vi "AerotechStateTransition.vi"(0 "error in (no error)":errorcluster, 5 "Command":T2, 7 "State In":T1) -> (3 "error out":errorcluster, 6 "Transition?":bool, 10 "State Out":T1)   [LabVIEW 2009]
uses:
  Controls/AerotechState.ctl
  Controls/AerotechCommand.ctl
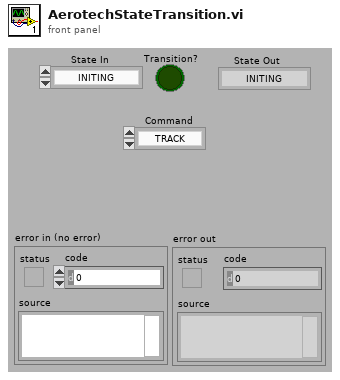
[diagram p1: front panel]
types:
  T1 = typedef "AerotechState.ctl" = enum16{"INITING", "IDLING", "SLEWING", "TRACKING", "MOVING", "HOMING", "STOPPING", "RECORDING"}
  T2 = typedef "AerotechCommand.ctl" = enum16{"TRACK", "POSITION", "STOP", "HOME", "QUIT", "RECORD"}
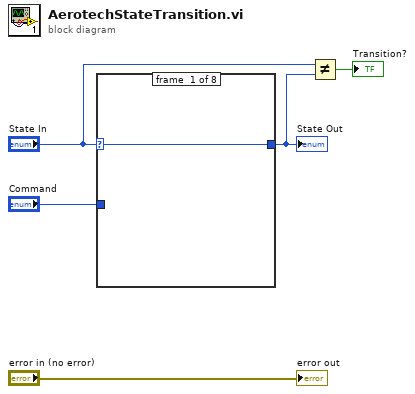
[diagram p0: block diagram]
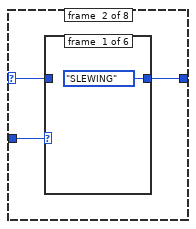
[diagram p2: hidden frame]
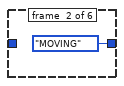
[diagram p3: hidden frame]
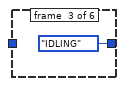
[diagram p4: hidden frame]
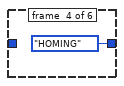
[diagram p5: hidden frame]
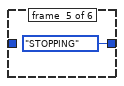
[diagram p6: hidden frame]
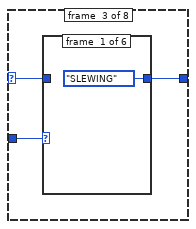
[diagram p8: hidden frame]
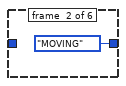
[diagram p9: hidden frame]
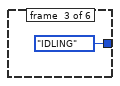
[diagram p10: hidden frame]
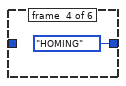
[diagram p11: hidden frame]
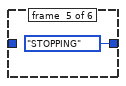
[diagram p12: hidden frame]
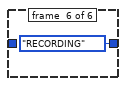
[diagram p13: hidden frame]
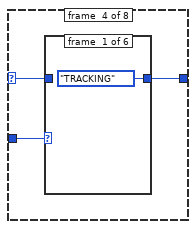
[diagram p14: hidden frame]
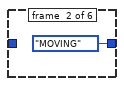
[diagram p15: hidden frame]
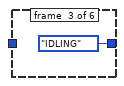
[diagram p16: hidden frame]
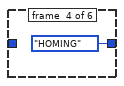
[diagram p17: hidden frame]
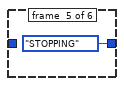
[diagram p18: hidden frame]
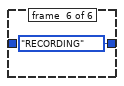
[diagram p19: hidden frame]
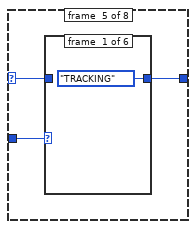
[diagram p20: hidden frame]
diagram:
  n1 = case shown="\"SLEWING\"" "State In" {
    selector: "State In" -> [w6 w7 w17 w26 w35 w44 w52 w53]
    tunnel: "Command" -> [_ w9 w18 w27 w36 w45 _ _]
    tunnel: [w6 w8 w16 w25 w34 w43 w52 w53] -> w3
    frame #0 {
    }
    frame #1 {
      n2 = case shown="\"TRACK\", Default" w9 {
        tunnel: [AerotechState."SLEWING" ("State In") AerotechState."MOVING" ("State In") AerotechState."IDLING" ("State In") AerotechState."HOMING" ("State In") AerotechState."STOPPING" ("State In") w15] -> w8
        tunnel: w7 -> [_ _ _ _ _ w15]
        frame #0 {
        }
        frame #1 {
        }
        frame #2 {
        }
        frame #3 {
        }
        frame #4 {
        }
        frame #5 {
        }
      }
    }
    frame #2 {
      n3 = case shown="\"RECORD\"" w18 {
        tunnel: w17 -> [_ _ _ _ _ _]
        tunnel: [AerotechState."SLEWING" ("State In") AerotechState."MOVING" ("State In") AerotechState."IDLING" ("State In") AerotechState."HOMING" ("State In") AerotechState."STOPPING" ("State In") AerotechState."RECORDING" ("State In")] -> w16
        frame #0 {
        }
        frame #1 {
        }
        frame #2 {
        }
        frame #3 {
        }
        frame #4 {
        }
        frame #5 {
        }
      }
    }
    frame #3 {
      n4 = case shown="\"RECORD\"" w27 {
        tunnel: w26 -> [_ _ _ _ _ _]
        tunnel: [AerotechState."TRACKING" ("State In") AerotechState."MOVING" ("State In") AerotechState."IDLING" ("State In") AerotechState."HOMING" ("State In") AerotechState."STOPPING" ("State In") AerotechState."RECORDING" ("State In")] -> w25
        frame #0 {
        }
        frame #1 {
        }
        frame #2 {
        }
        frame #3 {
        }
        frame #4 {
        }
        frame #5 {
        }
      }
    }
    frame #4 {
      n5 = case shown="\"RECORD\"" w36 {
        tunnel: w35 -> [_ _ _ _ _ w42]
        tunnel: [AerotechState."TRACKING" ("State In") AerotechState."MOVING" ("State In") AerotechState."IDLING" ("State In") AerotechState."HOMING" ("State In") AerotechState."STOPPING" ("State In") w42] -> w34
        frame #0 {
        }
        frame #1 {
        }
        frame #2 {
        }
        frame #3 {
        }
        frame #4 {
        }
        frame #5 {
        }
      }
    }
    frame #5 {
      n6 = case shown="\"RECORD\"" w45 {
        tunnel: w44 -> [w46 w47 w48 w49 _ w51]
        tunnel: [w46 w47 w48 w49 AerotechState."STOPPING" ("State In") w51] -> w43
        frame #0 {
        }
        frame #1 {
        }
        frame #2 {
        }
        frame #3 {
        }
        frame #4 {
        }
        frame #5 {
        }
      }
    }
    frame #6 {
    }
    frame #7 {
    }
  }
  "State Out" <- w3
  n7 = Not Equal?(x="State In", y=w3) -> (x != y?=→"Transition?":bool)
  "error out" <- "error in (no error)"
